vi "Set Switch HW Custom Device.vi"(8 "error in (no error)":errorcluster, 10 "Settings":T1, 11 "Switch HW Custom Device in":refnum<k24>) -> (0 "error out":errorcluster, 3 "Switch HW Custom Device out":refnum<k24>)   [LabVIEW 2017, in "Switch Scripting.lvlib"]
uses:
  Switch Scripting.lvlib
  Switch HW Custom Device Settings.ctl
  NationalInstruments.VeriStand.SystemDefinitionAPI
  <vilib>/NI VeriStand/Custom Device API/Custom Device API.lvlib
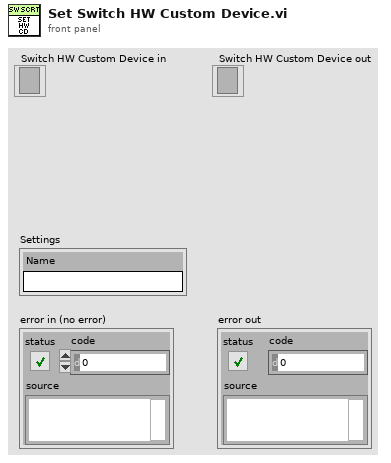
[diagram p1: front panel]
types:
  T1 = typedef "Switch Scripting.lvlib/Switch HW Custom Device Settings.ctl" = cluster{"Name":string}
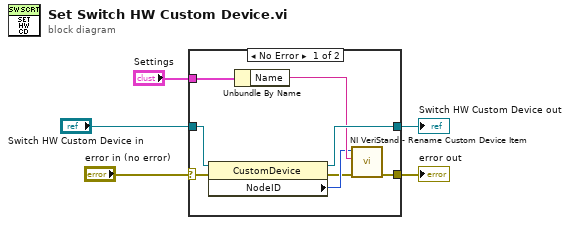
[diagram p0: block diagram]
diagram:
  n1 = case shown="No Error" "error in (no error)" {
    selector: "error in (no error)" -> [w11 w15]
    tunnel: "Settings" -> [w13 _]
    tunnel: [w6 w15] -> w4
    tunnel: [w12 w14] -> w3
    tunnel: "Switch HW Custom Device in" -> [w10 w14]
    frame No Error {
      n2 = property class="CustomDevice"(reference=w10, error in=w11) -> (reference out=w12:refnum<k24>, error out=w7:errorcluster, "NodeID"=w8:u64)
      n3 = Unbundle By Name(w13) -> ("Name"=w9:string)
      n4 = call <vilib>:"NI VeriStand - Rename Custom Device Item.vi"("error in (no error)"=w7, "New Name"=w9, "Item Ref in"=w8) -> ("error out"=w6:errorcluster)  [unwired: 6 in, 2 out]
    }
    frame Error {
    }
  }
  "error out" <- w4
  "Switch HW Custom Device out" <- w3
